vi "4ToF Playground.vi"() -> ()   [LabVIEW 2017]
uses:
  <vilib>/MakerHub/LINX/Public/Utilities/Open Local.vi
  Sensors/Time of Flight - VL6180/VL6180 states.ctl
  Sensors/Time of Flight - VL6180/VL6180 Resource.ctl
  <vilib>/MakerHub/LINX/Public/Peripherals/Digital/Digital Write 1 Chan.vi
panel:
  in  "Stop":bool
  in  "Wait (ms)":u32=10
  in  "Speed Read":bool
  out "Attempts":i32
  out "Sensor Error Code":u8
  in  "Attempts before Timeout":u16=10
  out "Gap 1":u8(slide) scale=0.0..100.0
  out "Rail Gap 1":u8(slide) scale=0.0..100.0
  out "Gap 2":u8(slide) scale=0.0..100.0
  out "Gap 3":u8(slide) scale=0.0..200.0
  out "Gap 4":u8(slide) scale=0.0..100.0
  out "Rail Gap 2":u8(slide) scale=0.0..100.0
  in  "delay":u32=100
  in  "I2C Channel":u8=1
  out "Sensors Online":bool[](array[boolean])
  in  "# of sensors":i32=5
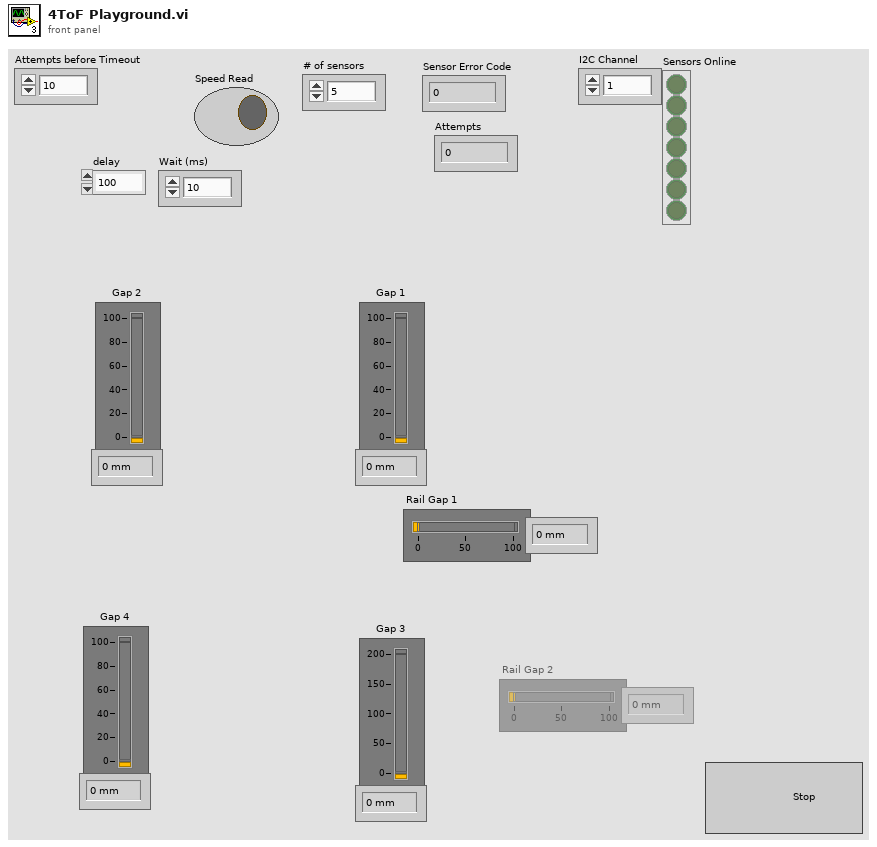
[diagram p1: front panel]
types:
  T1 = typedef "VL6180 states.ctl" = enum16{"Ping All", "Initialize", "Read"}
  T2 = typedef "LMH-LINX.lvlib/LINX Ref.ctl" = cluster{"IO":T3, "Interface":T4, "LINX Device Config":T5}
  T3 = typedef "LMH-LINX.lvlib/Platform.ctl" = enum16{"Remote", "Local"}
  T4 = typedef "LMH-LINX.lvlib/Interface.ctl" = enum16{"Serial", "TCP"}
  T5 = typedef "LMH-LINX.lvlib/Device.lvlib/LINX Device Config.ctl" = cluster{"Interface":T4, "COM Port":refnum<visa-resource-name>, "TCP Configuration":T6, "Device Family":u8, "Device ID":u8, "Device Name":string, "TCP Ref":refnum<k5>, "Channels":T7}
  T6 = typedef "LMH-LINX.lvlib/Device.lvlib/TCP Config.ctl" = cluster{"IP Address":string, "Port":u16}
  T7 = typedef "LMH-LINX.lvlib/Channels.ctl" = cluster{"DI":u8[], "DO":u8[], "AI":u8[], "AO":u8[], "PWM":u8[], "QE":u8[], "UART":u8[], "I2C 2":u8[], "SPI":u8[], "CAN":u8[], "Servo":u8[], "AI Ref (V)":dbl, "AI Resolution (Bits)":u8, "AO Ref (V)":dbl, "AO Resolution (Bits)":u8}
  T8 = typedef "VL6180 Resource.ctl" = cluster{"I2C Channel":u8, "I2C Slave Address":u8, "Online":bool}
  T9 = typedef "tofReading.ctl" = cluster{"Distance(mm)":u8, "Online":bool, "Error\nCode":u8, "Time Stamp":timestamp}
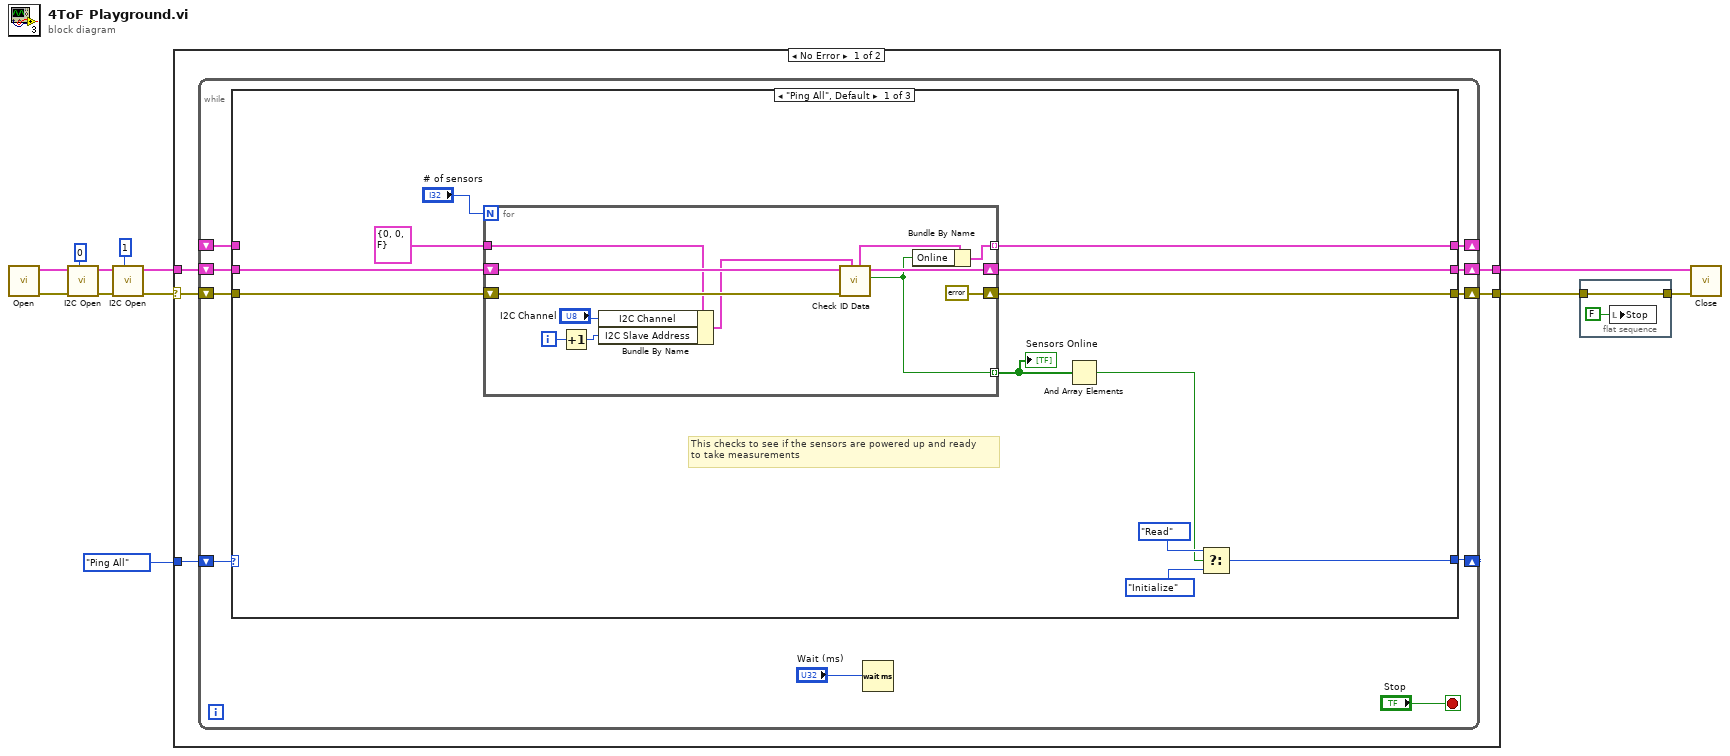
[diagram p0: block diagram]
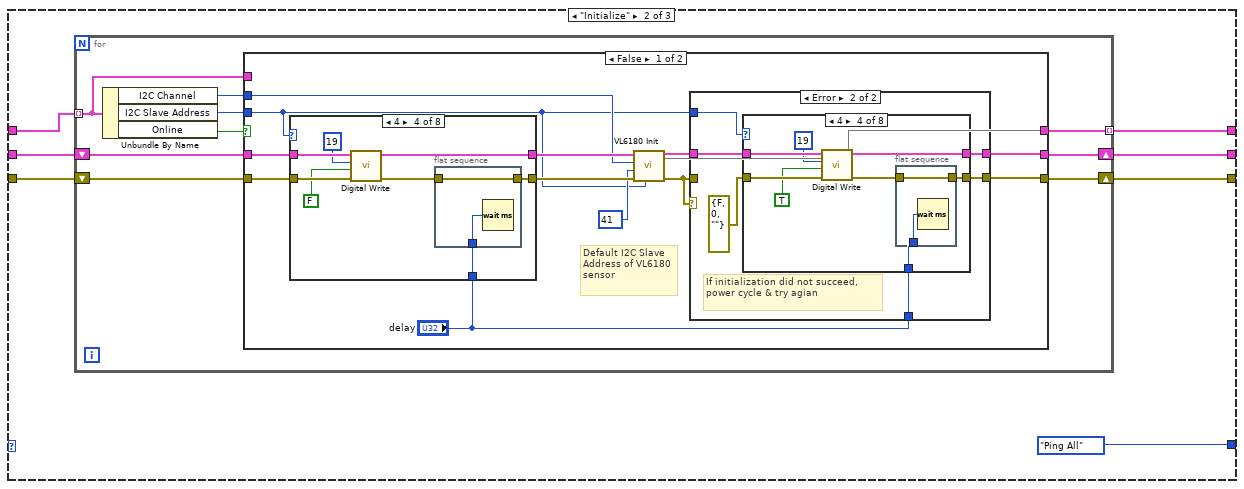
[diagram p2: hidden frame]
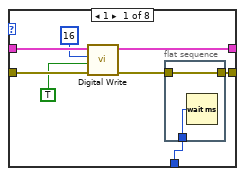
[diagram p4: hidden frame]
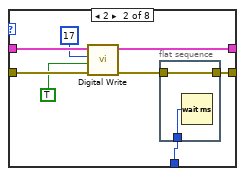
[diagram p5: hidden frame]
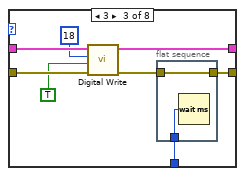
[diagram p6: hidden frame]
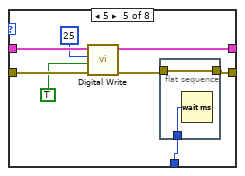
[diagram p7: hidden frame]
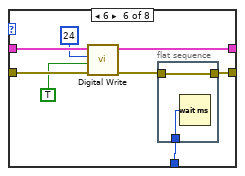
[diagram p8: hidden frame]
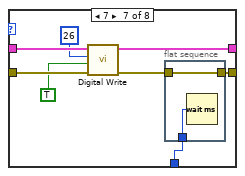
[diagram p9: hidden frame]
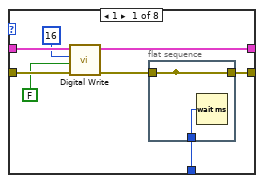
[diagram p11: hidden frame]
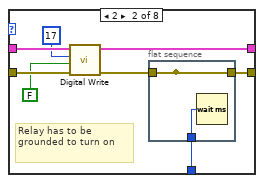
[diagram p12: hidden frame]
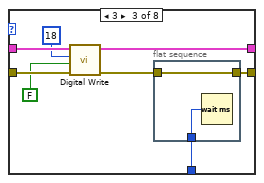
[diagram p13: hidden frame]
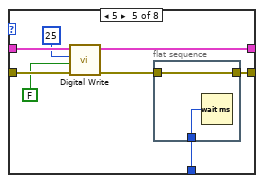
[diagram p14: hidden frame]
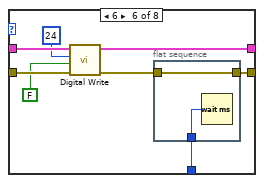
[diagram p15: hidden frame]
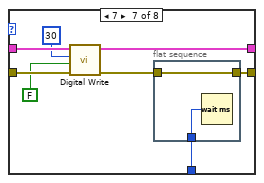
[diagram p16: hidden frame]
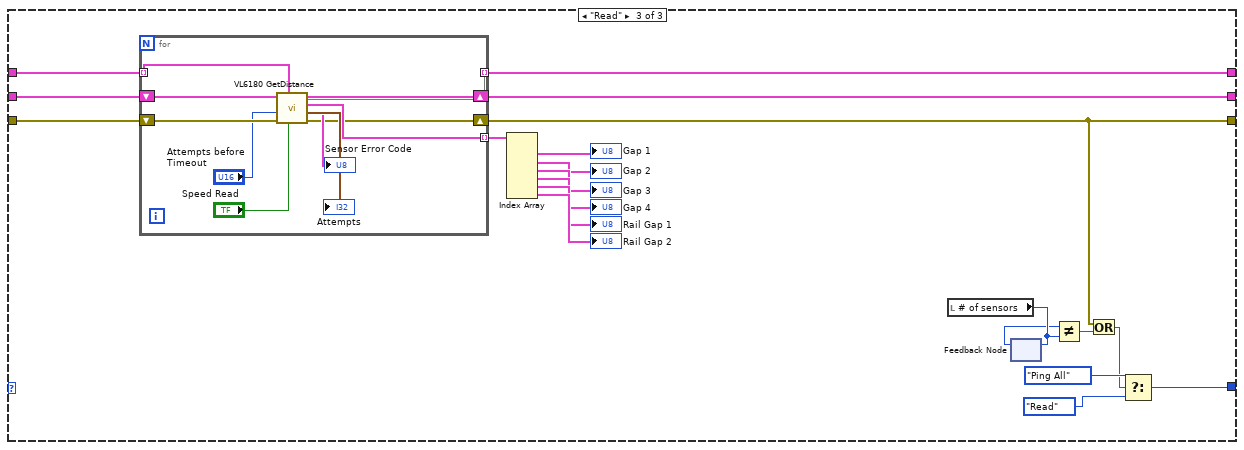
[diagram p19: hidden frame]
diagram:
  n1 = call-poly <vilib>:"Open.vi"() -> ("Error Out"=w5:errorcluster, "LINX Resource"=w6:T2)  [unwired: 9 in, 1 out]
  n2 = call <vilib>:"I2C Open.vi"("I2C Channel (0)"=u8 0, "Error In"=w5, "LINX Resource"=w6) -> ("Error Out"=w4:errorcluster, "LINX Resource"=w3:T2)  [unwired: 7 in]
  n3 = call <vilib>:"I2C Open.vi"("I2C Channel (0)"=u8 1, "Error In"=w4, "LINX Resource"=w3) -> ("Error Out"=w8:errorcluster, "LINX Resource"=w1:T2)  [unwired: 7 in]
  n4 = case shown="No Error" w8 {
    selector: w8 -> [w15 w268]
    tunnel: [w17 w268] -> w10
    tunnel: [w16 w267] -> w11
    tunnel: VL6180_states."Ping All" -> [w14 _]
    tunnel: w1 -> [w13 w267]
    frame No Error {
      n5 = while {
        shift-right: [w19] -> w16
        shift-left: w13 -> [w25]
        shift-right: [w18] -> w17
        shift-left: w15 -> [w24]
        shift-right: [w20] -> _
        shift-left: _ -> [w23]
        shift-right: [w21] -> _
        shift-left: w14 -> [w22]
        stop <- "Stop" stop-if-true
        n6 = case shown="\"Ping All\", Default" w22 {
          tunnel: w25 -> [w39 w58 w253]
          tunnel: w24 -> [w38 w52 w255]
          tunnel: w23 -> [_ w56 w252]
          tunnel: [w36 w53 w254] -> w20
          tunnel: [w37 w55 w248] -> w19
          tunnel: [w35 VL6180_states."Ping All" w251] -> w21
          tunnel: [w34 w54 w247] -> w18
          frame "Ping All", Default {
            # "This checks to see if the sensors are powered up and ready\nto take measurements"
            n7 = for {
              N: "# of sensors" -> [_]
              tunnel: T8 {"I2C Channel"=0, "I2C Slave Address"=0, "Online"=FALSE} ("VL6180 Resource out") -> [w44]
              shift-right: [w47] -> w37
              shift-left: w39 -> [w51]
              tunnel: [w46] -> w36 mode=indexing
              tunnel: [w45] -> w33 mode=indexing
              shift-right: [errorcluster {"status"=FALSE, "code"=0, "source"=""} ("error IO")] -> w34
              shift-left: w38 -> [w50]
              i -> [w48]
              n8 = Increment(x=w48) -> (x+1=w41:i32)
              n9 = Bundle By Name(cluster=w44, "I2C Channel"="I2C Channel", "I2C Slave Address"=w41) -> (w43:T8)
              n10 = call "Check ID Data.vi"("VL6180 Resource"=w43, "Error In"=w50, "LINX Resource"=w51) -> ("Same Model?"=w45:bool, "LINX Resource"=w47:T2, "VL6180 Resource"=w49:T8)  [unwired: 5 in, 1 out]
              n11 = Bundle By Name(cluster=w49, "Online"=w45) -> (w46:T8)
            }
            "Sensors Online" <- w33
            n12 = And Array Elements(Boolean array=w33) -> (logical AND=w30:bool)
            n13 = Select(t=VL6180_states."Read", s=w30, f=VL6180_states."Initialize") -> (s? t:f=w35:T1)
          }
          frame "Initialize" {
            n14 = for {
              tunnel: w56 -> [w59] mode=indexing
              shift-right: [w66] -> w55
              shift-left: w58 -> [w67]
              shift-right: [w65] -> w54
              shift-left: w52 -> [w61]
              tunnel: [w62] -> w53 mode=indexing
              n15 = Unbundle By Name(w59) -> ("I2C Channel"=w64:u8, "I2C Slave Address"=w63:u8, "Online"=w60:bool)
              n16 = case shown="False" w60 {
                tunnel: w67 -> [w80 w235]
                tunnel: w61 -> [w77 w234]
                tunnel: [w74 w235] -> w66
                tunnel: [w73 w234] -> w65
                tunnel: w64 -> [w69 _]
                tunnel: w63 -> [w68 _]
                tunnel: [w75 w233] -> w62
                tunnel: w59 -> [_ w233]
                frame False {
                  # "Default I2C Slave Address of VL6180 sensor"
                  n17 = case shown="4" w68 {
                    tunnel: w80 -> [w168 w178 w188 w198 w208 w218 w228 w232]
                    tunnel: [w167 w177 w187 w197 w207 w217 w227 w232] -> w79
                    tunnel: [w163 w173 w182 w192 w202 w212 w222 w231] -> w78
                    tunnel: w77 -> [w166 w176 w186 w196 w206 w216 w226 w231]
                    tunnel: "delay" -> [w161 w171 w181 w191 w201 w211 w221 _]
                    frame 1 {
                      n18 = call-poly <vilib>:"Digital Write.vi"("Error In"=w166, "Output Value"=FALSE, "DO Channel"=u8 16, "LINX Resource"=w168) -> ("Error Out"=w162:errorcluster, "LINX Resource"=w167:T2)  [unwired: 6 in]
                      n19 = flat-sequence {
                        tunnel: [w170] -> _
                        tunnel: [w170] -> w163
                        tunnel: w162 -> [w170]
                        tunnel: w161 -> [w169]
                        frame #0 {
                          n20 = Wait (ms)(milliseconds to wait=w169) -> ()  [unwired: 1 out]
                        }
                      }
                    }
                    frame 2 {
                      # "Relay has to be grounded to turn on"
                      n21 = call-poly <vilib>:"Digital Write.vi"("Error In"=w176, "Output Value"=FALSE, "DO Channel"=u8 17, "LINX Resource"=w178) -> ("Error Out"=w172:errorcluster, "LINX Resource"=w177:T2)  [unwired: 6 in]
                      n22 = flat-sequence {
                        tunnel: [w180] -> _
                        tunnel: [w180] -> w173
                        tunnel: w172 -> [w180]
                        tunnel: w171 -> [w179]
                        frame #0 {
                          n23 = Wait (ms)(milliseconds to wait=w179) -> ()  [unwired: 1 out]
                        }
                      }
                    }
                    frame 3 {
                      n24 = call-poly <vilib>:"Digital Write.vi"("Error In"=w186, "Output Value"=FALSE, "DO Channel"=u8 18, "LINX Resource"=w188) -> ("Error Out"=w183:errorcluster, "LINX Resource"=w187:T2)  [unwired: 6 in]
                      n25 = flat-sequence {
                        tunnel: w183 -> [w190]
                        tunnel: [w190] -> w182
                        tunnel: w181 -> [w189]
                        frame #0 {
                          n26 = Wait (ms)(milliseconds to wait=w189) -> ()  [unwired: 1 out]
                        }
                      }
                    }
                    frame 4 {
                      n27 = call-poly <vilib>:"Digital Write.vi"("Error In"=w196, "Output Value"=FALSE, "DO Channel"=u8 19, "LINX Resource"=w198) -> ("Error Out"=w193:errorcluster, "LINX Resource"=w197:T2)  [unwired: 6 in]
                      n28 = flat-sequence {
                        tunnel: w193 -> [w200]
                        tunnel: [w200] -> w192
                        tunnel: w191 -> [w199]
                        frame #0 {
                          n29 = Wait (ms)(milliseconds to wait=w199) -> ()  [unwired: 1 out]
                        }
                      }
                    }
                    frame 5 {
                      n30 = call-poly <vilib>:"Digital Write.vi"("Error In"=w206, "Output Value"=FALSE, "DO Channel"=u8 25, "LINX Resource"=w208) -> ("Error Out"=w203:errorcluster, "LINX Resource"=w207:T2)  [unwired: 6 in]
                      n31 = flat-sequence {
                        tunnel: w203 -> [w210]
                        tunnel: [w210] -> w202
                        tunnel: w201 -> [w209]
                        frame #0 {
                          n32 = Wait (ms)(milliseconds to wait=w209) -> ()  [unwired: 1 out]
                        }
                      }
                    }
                    frame 6 {
                      n33 = call-poly <vilib>:"Digital Write.vi"("Error In"=w216, "Output Value"=FALSE, "DO Channel"=u8 24, "LINX Resource"=w218) -> ("Error Out"=w213:errorcluster, "LINX Resource"=w217:T2)  [unwired: 6 in]
                      n34 = flat-sequence {
                        tunnel: w213 -> [w220]
                        tunnel: [w220] -> w212
                        tunnel: w211 -> [w219]
                        frame #0 {
                          n35 = Wait (ms)(milliseconds to wait=w219) -> ()  [unwired: 1 out]
                        }
                      }
                    }
                    frame 7 {
                      n36 = call-poly <vilib>:"Digital Write.vi"("Error In"=w226, "Output Value"=FALSE, "DO Channel"=u8 30, "LINX Resource"=w228) -> ("Error Out"=w223:errorcluster, "LINX Resource"=w227:T2)  [unwired: 6 in]
                      n37 = flat-sequence {
                        tunnel: w223 -> [w230]
                        tunnel: [w230] -> w222
                        tunnel: w221 -> [w229]
                        frame #0 {
                          n38 = Wait (ms)(milliseconds to wait=w229) -> ()  [unwired: 1 out]
                        }
                      }
                    }
                    frame 9, Default {
                    }
                  }
                  n39 = call "VL6180 Init.vi"("Change Slave Address"=w68, "Error In"=w78, "I2C Slave Address"=u8 41 ("I2C Slave Address (0)"), "I2C Channel"=w69, "LINX Resource"=w79) -> ("Error Out"=w71:errorcluster, "LINX Resource"=w72:T2, 5:w75)  [unwired: 3 in, 1 out]
                  n40 = case shown="Error" w71 {
                    tunnel: [w82 w88] -> w74
                    tunnel: [w81 w85] -> w73
                    tunnel: w72 -> [w82 w87]
                    tunnel: w71 -> [w81 _]
                    tunnel: "delay" -> [_ w84]
                    tunnel: w68 -> [_ w83]
                    frame No Error {
                      # "Initialization successful"
                    }
                    frame Error {
                      # "If initialization did not succeed, power cycle & try agian"
                      n41 = case shown="4" w83 {
                        tunnel: w87 -> [w96 w106 w116 w126 w136 w146 w156 w160]
                        tunnel: [w95 w105 w115 w125 w135 w145 w155 w160] -> w88
                        tunnel: [w90 w99 w110 w120 w130 w140 w150 w159] -> w85
                        tunnel: errorcluster {"status"=FALSE, "code"=0, "source"=""} ("Error Out") -> [w94 w104 w114 w124 w134 w144 w154 w159]
                        tunnel: w84 -> [w89 w100 w109 w119 w129 w139 w149 _]
                        frame 1 {
                          n42 = call-poly <vilib>:"Digital Write.vi"("Error In"=w94, "Output Value"=TRUE, "DO Channel"=u8 16, "LINX Resource"=w96) -> ("Error Out"=w91:errorcluster, "LINX Resource"=w95:T2)  [unwired: 6 in]
                          n43 = flat-sequence {
                            tunnel: [w98] -> w90
                            tunnel: w91 -> [w98]
                            tunnel: w89 -> [w97]
                            frame #0 {
                              n44 = Wait (ms)(milliseconds to wait=w97) -> ()  [unwired: 1 out]
                            }
                          }
                        }
                        frame 2 {
                          n45 = call-poly <vilib>:"Digital Write.vi"("Error In"=w104, "Output Value"=TRUE, "DO Channel"=u8 17, "LINX Resource"=w106) -> ("Error Out"=w101:errorcluster, "LINX Resource"=w105:T2)  [unwired: 6 in]
                          n46 = flat-sequence {
                            tunnel: [w108] -> w99
                            tunnel: w101 -> [w108]
                            tunnel: w100 -> [w107]
                            frame #0 {
                              n47 = Wait (ms)(milliseconds to wait=w107) -> ()  [unwired: 1 out]
                            }
                          }
                        }
                        frame 3 {
                          n48 = call-poly <vilib>:"Digital Write.vi"("Error In"=w114, "Output Value"=TRUE, "DO Channel"=u8 18, "LINX Resource"=w116) -> ("Error Out"=w111:errorcluster, "LINX Resource"=w115:T2)  [unwired: 6 in]
                          n49 = flat-sequence {
                            tunnel: [w118] -> w110
                            tunnel: w111 -> [w118]
                            tunnel: w109 -> [w117]
                            frame #0 {
                              n50 = Wait (ms)(milliseconds to wait=w117) -> ()  [unwired: 1 out]
                            }
                          }
                        }
                        frame 4 {
                          n51 = call-poly <vilib>:"Digital Write.vi"("Error In"=w124, "Output Value"=TRUE, "DO Channel"=u8 19, "LINX Resource"=w126) -> ("Error Out"=w121:errorcluster, "LINX Resource"=w125:T2)  [unwired: 6 in]
                          n52 = flat-sequence {
                            tunnel: [w128] -> w120
                            tunnel: w121 -> [w128]
                            tunnel: w119 -> [w127]
                            frame #0 {
                              n53 = Wait (ms)(milliseconds to wait=w127) -> ()  [unwired: 1 out]
                            }
                          }
                        }
                        frame 5 {
                          n54 = call-poly <vilib>:"Digital Write.vi"("Error In"=w134, "Output Value"=TRUE, "DO Channel"=u8 25, "LINX Resource"=w136) -> ("Error Out"=w131:errorcluster, "LINX Resource"=w135:T2)  [unwired: 6 in]
                          n55 = flat-sequence {
                            tunnel: [w138] -> w130
                            tunnel: w131 -> [w138]
                            tunnel: w129 -> [w137]
                            frame #0 {
                              n56 = Wait (ms)(milliseconds to wait=w137) -> ()  [unwired: 1 out]
                            }
                          }
                        }
                        frame 6 {
                          n57 = call-poly <vilib>:"Digital Write.vi"("Error In"=w144, "Output Value"=TRUE, "DO Channel"=u8 24, "LINX Resource"=w146) -> ("Error Out"=w141:errorcluster, "LINX Resource"=w145:T2)  [unwired: 6 in]
                          n58 = flat-sequence {
                            tunnel: [w148] -> w140
                            tunnel: w141 -> [w148]
                            tunnel: w139 -> [w147]
                            frame #0 {
                              n59 = Wait (ms)(milliseconds to wait=w147) -> ()  [unwired: 1 out]
                            }
                          }
                        }
                        frame 7 {
                          n60 = call-poly <vilib>:"Digital Write.vi"("Error In"=w154, "Output Value"=TRUE, "DO Channel"=u8 26, "LINX Resource"=w156) -> ("Error Out"=w151:errorcluster, "LINX Resource"=w155:T2)  [unwired: 6 in]
                          n61 = flat-sequence {
                            tunnel: [w158] -> w150
                            tunnel: w151 -> [w158]
                            tunnel: w149 -> [w157]
                            frame #0 {
                              n62 = Wait (ms)(milliseconds to wait=w157) -> ()  [unwired: 1 out]
                            }
                          }
                        }
                        frame 9, Default {
                        }
                      }
                    }
                  }
                }
                frame True {
                }
              }
            }
          }
          frame "Read" {
            n63 = for {
              tunnel: [w262] -> w254 mode=indexing
              shift-right: [w260] -> w248
              shift-left: w253 -> [w261]
              tunnel: w252 -> [w256] mode=indexing
              tunnel: [w259] -> w241 mode=indexing
              shift-right: [w258] -> w247
              shift-left: w255 -> [w266]
              n64 = call "VL6180 GetDistance.vi"("Speed Read"="Speed Read", 7:w256, "error in (no error)"=w266, "Attempts before Timeout"="Attempts before Timeout", "LINX Resource"=w261) -> ("error out"=w258:errorcluster, "ToF Reading"=→"Sensor Error Code":T9, "VL6180 Resource out"=w259:T8, "LINX Resource"=w260:T2, "VL6180 Error"=→"Attempts":cluster{"Error Code":u8, "# attempts":i32}, 5:w262)  [unwired: 1 in]
            }
            n65 = Index Array(array=w241) -> (element #1=→"Gap 1":T8, element #2=→"Gap 2":T8, element #3=→"Gap 3":T8, element #4=→"Gap 4":T8, element #5=→"Rail Gap 1":T8, element #6=→"Rail Gap 2":T8)  [unwired: 6 in]
            n66 = local read "# of sensors"() -> (w245:i32)
            n67 = feedback-in #1(w245) -> ()
            n68 = feedback #1() -> (w244:i32)  [unwired: 1 in]
            n69 = Not Equal?(x=w244, y=w245) -> (x != y?=w246:bool)
            n70 = Or(x=w247, y=w246) -> (x .or. y?=w243:bool)
            n71 = Select(t=VL6180_states."Ping All", s=w243, f=VL6180_states."Read") -> (s? t:f=w251:T1)
          }
        }
        n72 = Wait (ms)(milliseconds to wait="Wait (ms)") -> ()  [unwired: 1 out]
      }
    }
    frame Error {
    }
  }
  n73 = flat-sequence {
    tunnel: w10 -> [w269]
    tunnel: [w269] -> w9
    frame #0 {
      n74 = local write "Stop"(FALSE ("Stop")) -> ()
    }
  }
  n75 = call <vilib>:"Close.vi"("Error In"=w9, "LINX Resource"=w11) -> ()  [unwired: 9 in, 1 out]
